vi "SetSessionAction.vi"(8 "error in (no error)":errorcluster, 9 "ActionValue (False)":string[](array[string])=["False"], 10 "ActionName  (ForceField)":string[](array[string])) -> (0 "error out":errorcluster)   [LabVIEW 2016]
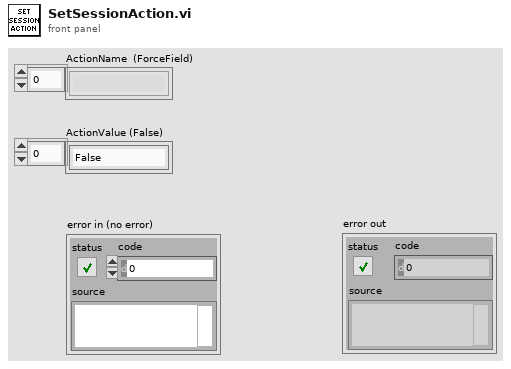
[diagram p1: front panel]
types:
  T1 = enum32{"Invalid", "Standard", "Closed", "Hidden", "Minimized", "Maximized"}
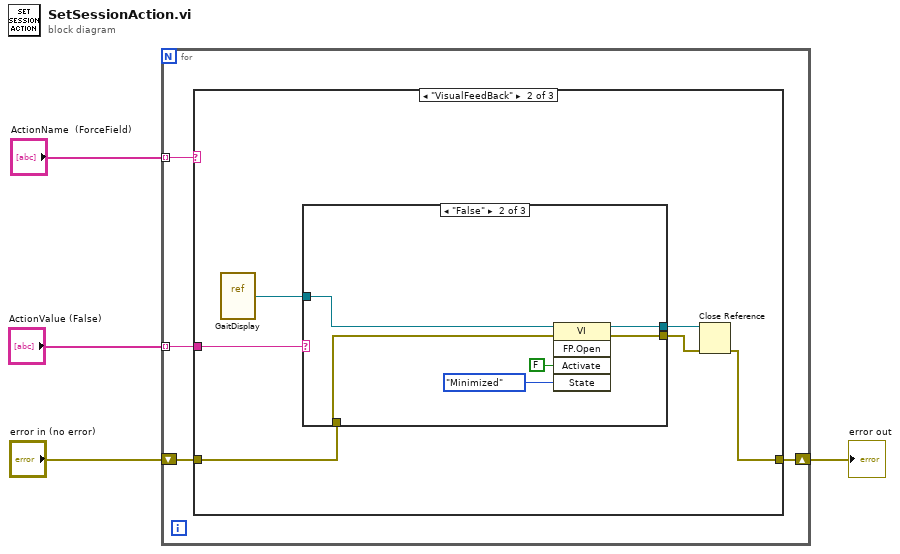
[diagram p0: block diagram]
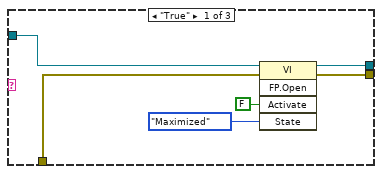
[diagram p3: hidden frame]
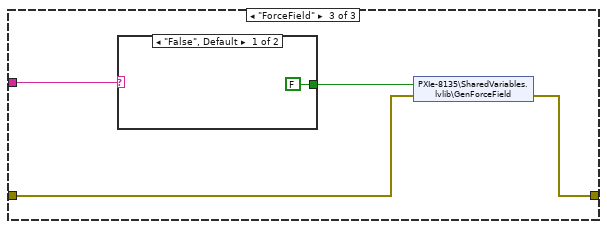
[diagram p5: hidden frame]
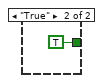
[diagram p6: hidden frame]
diagram:
  n1 = for {
    tunnel: "ActionName  (ForceField)" -> [w8] mode=indexing
    tunnel: "ActionValue (False)" -> [w7] mode=indexing
    shift-right: [w5] -> w1
    shift-left: "error in (no error)" -> [w6]
    n2 = case shown="\"VisualFeedBack\"" w8 {
      tunnel: w7 -> [_ w15 w33]
      tunnel: w6 -> [w9 w13 w31]
      tunnel: [w9 w11 w30] -> w5
      frame Default {
      }
      frame "VisualFeedBack" {
        n3 = vi-ref "GaitDisplay.vi"() -> (w14:refnum<vi>)
        n4 = case shown="\"False\"" w15 {
          tunnel: w14 -> [w21 w27 w28]
          tunnel: w13 -> [w20 w26 w29]
          tunnel: [w19 w25 w29] -> w12
          tunnel: [w18 w24 w28] -> w10
          frame "True" {
            n5 = invoke class="VI" method="FP.Open"(reference=w21, error in=w20, "Activate"=FALSE ("Activate?"), "State"=T1."Maximized") -> (reference out=w18:refnum<vi>, error out=w19:errorcluster)  [unwired: 1 in, 3 out]
          }
          frame "False" {
            n6 = invoke class="VI" method="FP.Open"(reference=w27, error in=w26, "Activate"=FALSE ("Activate?"), "State"=T1."Minimized") -> (reference out=w24:refnum<vi>, error out=w25:errorcluster)  [unwired: 1 in, 3 out]
          }
          frame Default {
          }
        }
        n7 = Close Reference(reference=w10, error in (no error)=w12) -> (error out=w11:errorcluster)
      }
      frame "ForceField" {
        n8 = case shown="\"False\", Default" w33 {
          tunnel: [FALSE TRUE] -> w32
          frame "False", Default {
          }
          frame "True" {
          }
        }
        n9 = shared-variable "PXIe-8135\\SharedVariables.lvlib\\GenForceField"(w32, error in=w31) -> (error out=w30:errorcluster)
      }
    }
  }
  "error out" <- w1
